vi "Test Impedance Data.vi"() -> ()   [LabVIEW 2019]
uses:
  <vilib>/Analysis/3filter.llb/Filter Passband Type.ctl
  <vilib>/Analysis/5stat.llb/RMS (DBL).vi
  <vilib>/Utility/file.llb/Read Delimited Spreadsheet (DBL).vi
  <vilib>/Analysis/3filter.llb/Butterworth Filter (DBL).vi
  <vilib>/Analysis/NI_AALPro.lvlib
  <vilib>/Analysis/NI_AALBase.lvlib
  <vilib>/ptbypt/NI_PtbyPt.lvlib
panel:
  out "Impedance in Ohm":dbl[](graph)
  out "Original Data Full":dbl[](graph)
  out "Filtered Data Full":dbl[](graph)
  in  "Boolean":bool=TRUE
  in  "ch":i32=1
  out "rms value":dbl format="%.7f"
  out "filtered data":dbl[](graph)
  out "original data":dbl[](graph)
  # "Unfilt"
  # "Filt"
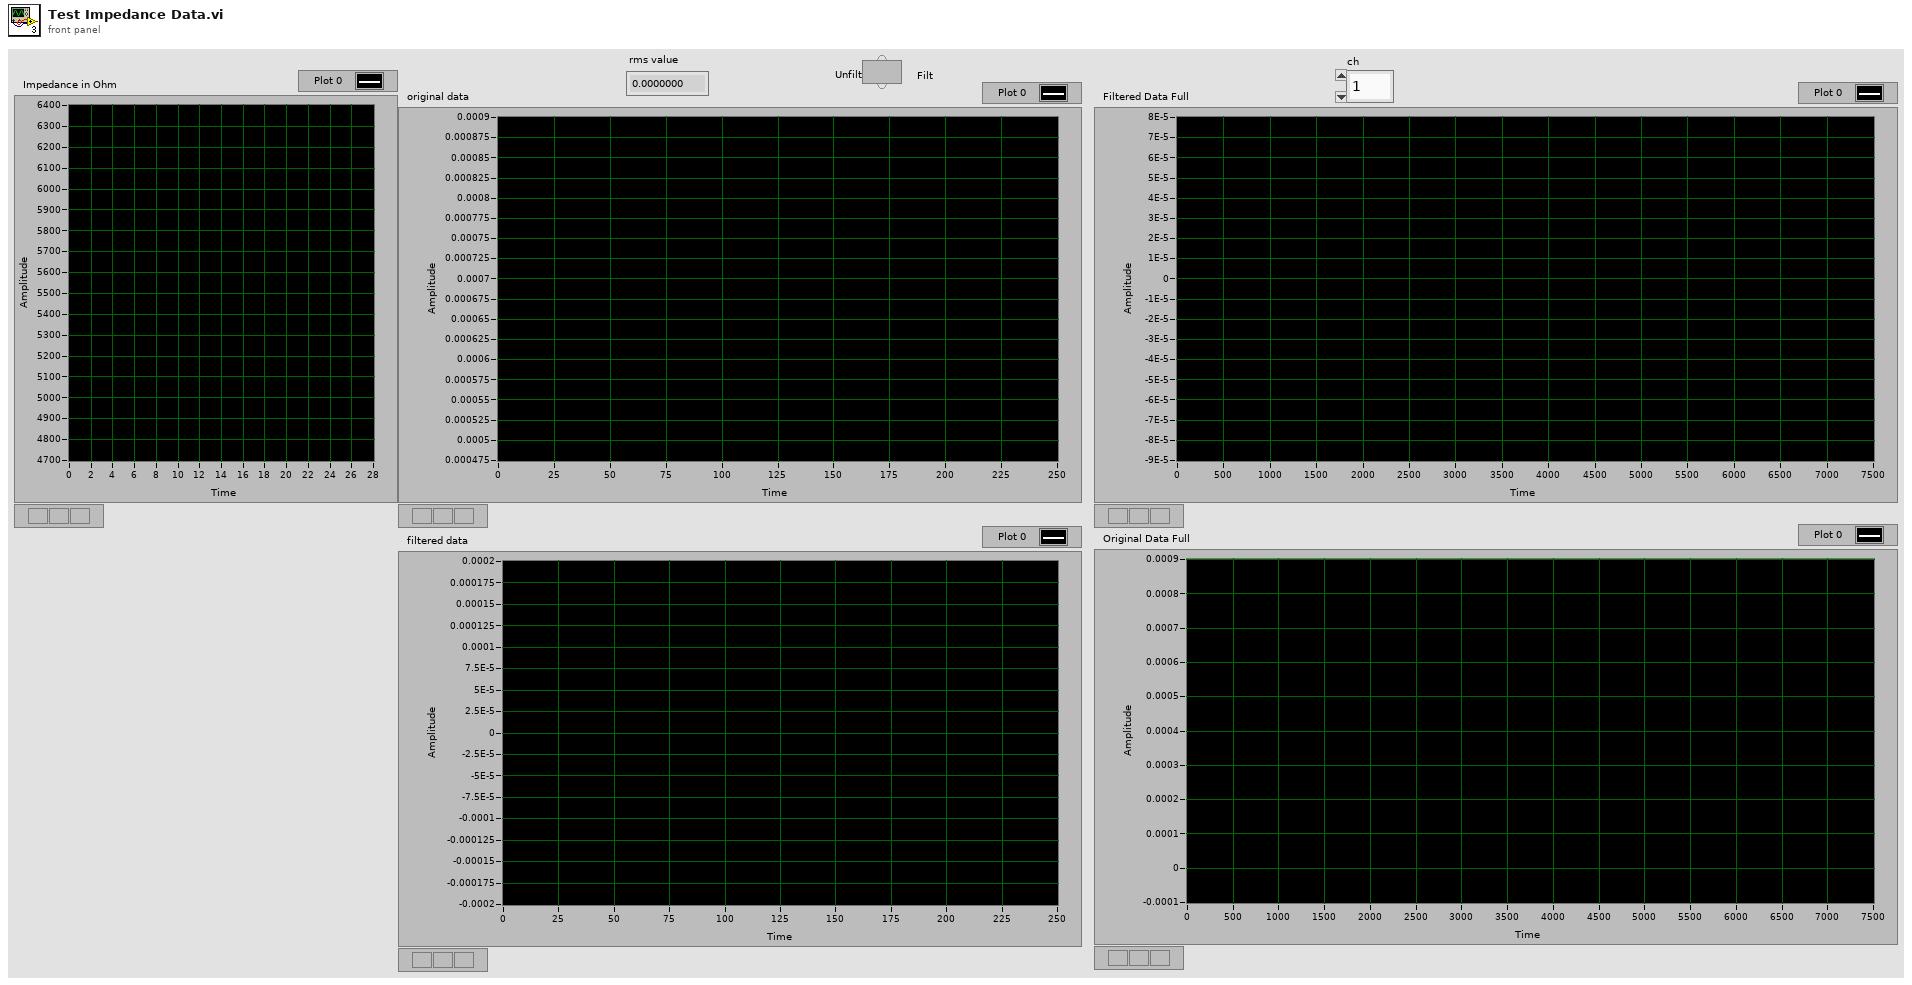
[diagram p1: front panel]
types:
  T1 = typedef "NI_AALBase.lvlib/Filter Passband Type.ctl" = enum32{"Lowpass", "Highpass", "Bandpass", "Bandstop"}
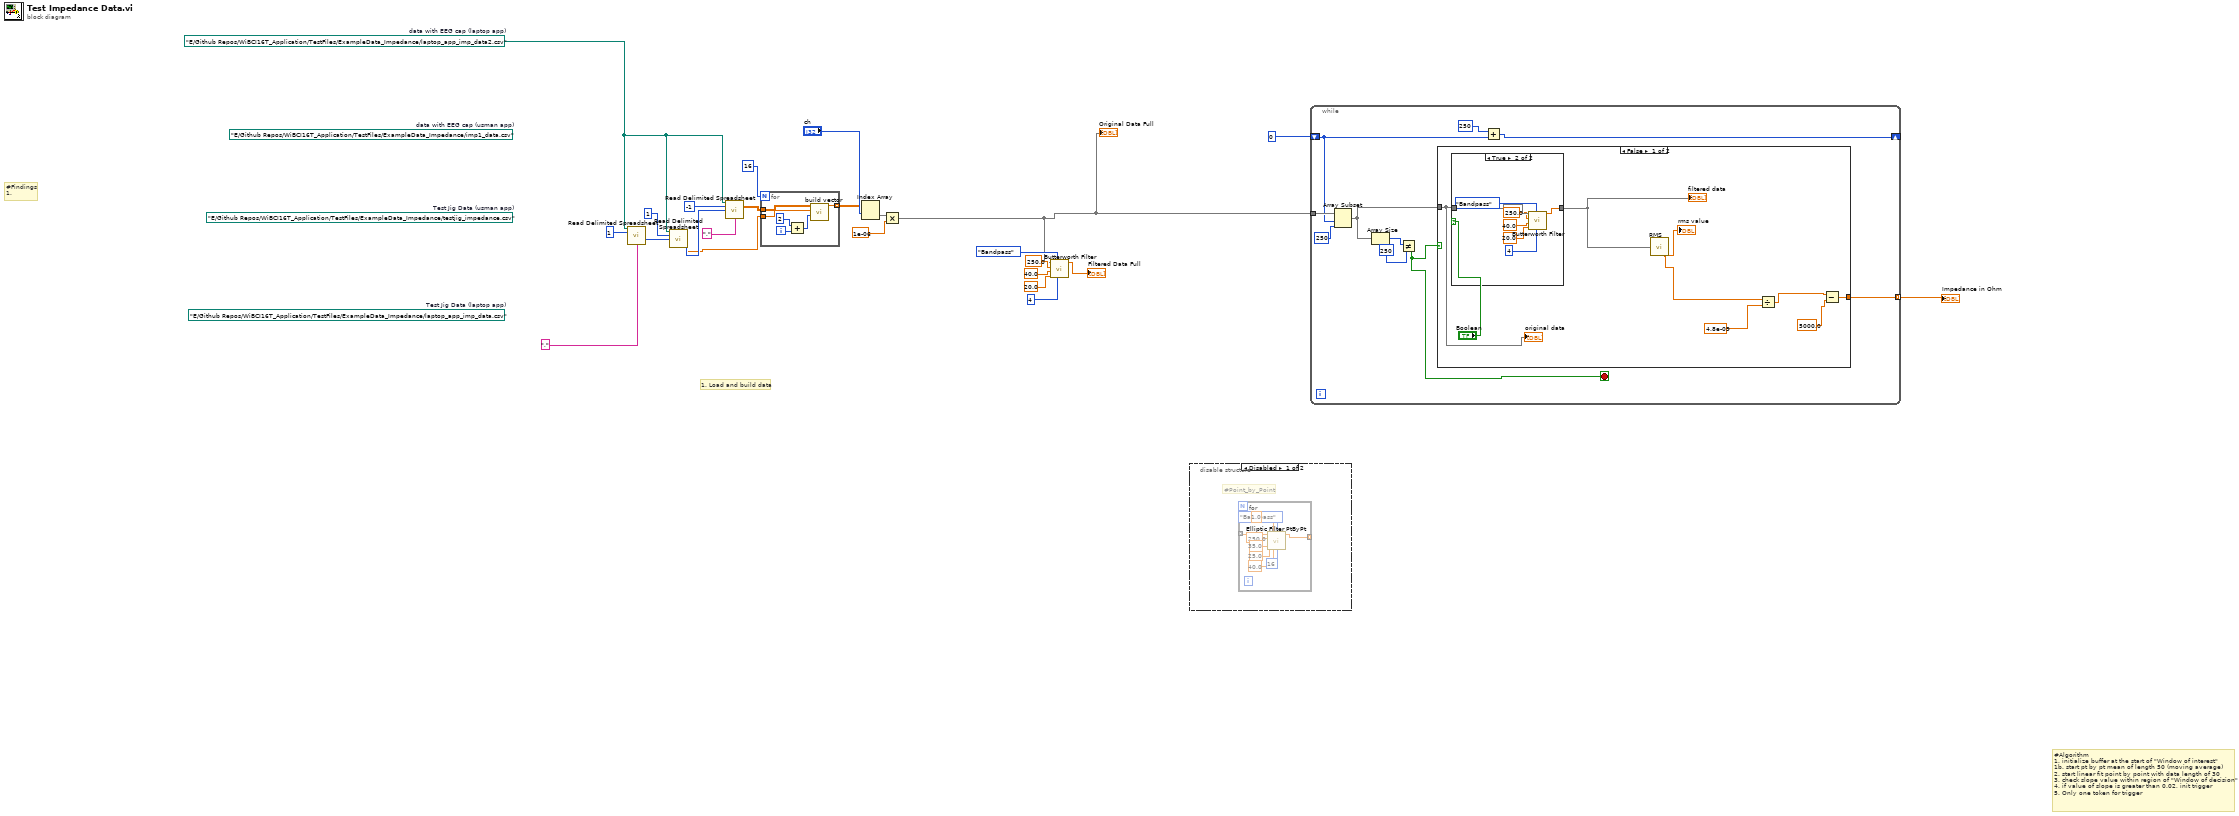
[diagram p0: block diagram]
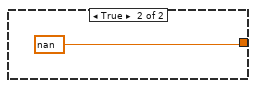
[diagram p4: hidden frame]
diagram:
  w1 = path "E:/Github Repos/WiBCI16T_Application/TestFiles/ExampleData_Impedance/laptop_app_imp_data2.csv"  # data with EEG cap (laptop app)
  (unwired) path "E:/Github Repos/WiBCI16T_Application/TestFiles/ExampleData_Impedance/laptop_app_imp_data.csv"  # Test Jig Data (laptop app)
  (unwired) path "E:/Github Repos/WiBCI16T_Application/TestFiles/ExampleData_Impedance/testjig_impedance.csv"  # Test Jig Data (usman app)
  (unwired) path "E:/Github Repos/WiBCI16T_Application/TestFiles/ExampleData_Impedance/imp1_data.csv"  # data with EEG cap (usman app)
  # "#Findings\n1."
  # "1. Load and build data"
  # "#Algorithm\n1. initialize buffer at the start of \"Window of interest\"\n1b. start pt by pt mean of length 50 (moving average)\n2. start linear fit point by point with data length of 30\n3. check slope value within region of \"Window of decision\"\n4. if value of slope is greater than 0.02, init trigger\n5. Only one token for trigger"
  n1 = call-poly <vilib>:"Read Delimited Spreadsheet.vi"("file path (dialog if empty)"=w1, "number of rows (all:-1)"=1, "delimiter (\\t)"=",") -> ("mark after read (chars.)"=w22:i32)  [unwired: 7 in, 5 out]
  n2 = call-poly <vilib>:"Read Delimited Spreadsheet.vi"("file path (dialog if empty)"=w1, "number of rows (all:-1)"=1, "start of read offset (chars.:0)"=w22) -> ("first row"=w9:dbl[], "mark after read (chars.)"=w16:i32)  [unwired: 7 in, 4 out]
  n3 = call-poly <vilib>:"Read Delimited Spreadsheet.vi"("file path (dialog if empty)"=w1, "number of rows (all:-1)"=-1, "start of read offset (chars.:0)"=w16, "delimiter (\\t)"=",") -> ("all rows"=w19:dbl[][])  [unwired: 6 in, 5 out]
  n4 = for {
    N: 16 -> [_]
    tunnel: w19 -> [w30]
    tunnel: w9 -> [w29]
    tunnel: [w25] -> w14 mode=indexing
    i -> [w28]
    n5 = Add(x=2, y=w28) -> (x+y=w26:i32)
    n6 = call "build vector.vi"("Index"=w26, "first row"=w29, "diff data"=w30) -> ("Rebuild Vector"=w25:dbl[])  [unwired: 8 in]
  }
  n7 = Index Array(array=w14, index (row)="ch") -> (element=w12:dbl[])  [unwired: 1 in]
  n8 = Multiply(x=w12, y=1e-06) -> (x*y=w3:dbl[])
  "Original Data Full" <- w3
  n9 = call-poly <vilib>:"Butterworth Filter.vi"("order"=4, "filter type"=Filter_Passband_Type."Bandpass", "low cutoff freq: fl"=20.0, "high cutoff freq: fh"=40.0, "sampling freq: fs"=250.0, "X"=w3) -> ("Filtered X"=→"Filtered Data Full":dbl[])  [unwired: 2 in, 1 out]
  n10 = disable-structure shown="Disabled" {
    frame Disabled {
      # "#Point_by_Point"
      n11 = for {
        tunnel: _ -> [w39] mode=indexing
        tunnel: [w33] -> _ mode=indexing
        n12 = call <vilib>:"Elliptic Filter PtByPt.vi"("x"=w39, "passband ripple (dB)"=1.0, "filter type"=Filter_Passband_Type."Bandpass", "sampling freq: fs"=250.0, "high cutoff freq: fh"=35.0, "low cutoff freq: fl"=25.0, "stopband attenuation(dB)"=40.0, "order"=16) -> ("Filtered x"=w33:dbl)  [unwired: 6 in, 1 out]
      }
    }
    frame Enabled {
    }
  }
  n13 = while {
    tunnel: w3 -> [w49]
    shift-right: [w47] -> _
    shift-left: 0 -> [w48]
    tunnel: [w40] -> w10 mode=indexing
    stop <- w42 stop-if-true
    n14 = Array Subset(array=w49, index=w48, length=250) -> (w41:dbl[])
    n15 = Array Size(array=w41) -> (size(s)=w44:i32)
    n16 = Not Equal?(x=w44, y=250) -> (x != y?=w42:bool)
    n17 = case shown="False" w42 {
      tunnel: w41 -> [w50 _]
      tunnel: [w56 nan] -> w40
      frame False {
        n18 = case shown="True" "Boolean" {
          tunnel: w50 -> [w58 w65]
          tunnel: [w58 w64] -> w52
          frame False {
          }
          frame True {
            n19 = call-poly <vilib>:"Butterworth Filter.vi"("order"=4, "filter type"=Filter_Passband_Type."Bandpass", "low cutoff freq: fl"=20.0, "high cutoff freq: fh"=40.0, "sampling freq: fs"=250.0, "X"=w65) -> ("Filtered X"=w64:dbl[])  [unwired: 2 in, 1 out]
          }
        }
        "filtered data" <- w52
        n20 = call-poly <vilib>:"RMS.vi"("X"=w52) -> ("rms value"=w57:dbl)  [unwired: 1 out]
        "rms value" <- w57
        n21 = Divide(x=w57, y=4.8e-09) -> (x/y=w54:dbl)
        n22 = Subtract(x=w54, y=5000.0) -> (x-y=w56:dbl)
        "original data" <- w50
      }
      frame True {
      }
    }
    n23 = Add(x=250, y=w48) -> (x+y=w47:i32)
  }
  "Impedance in Ohm" <- w10
